vi "Start Sync.vi"(8 "error in (no error)":errorcluster, 11 "gRPC service in":refnum<class "OOBgRPCService.lvclass">) -> (0 "error out":errorcluster, 3 "gRPC service out":refnum<class "OOBgRPCService.lvclass">)   [LabVIEW 2025, in "OOB gRPC Server.lvlib" / "OOBgRPCService.lvclass"]
uses:
  OOBgRPCService.lvclass
  OOBgRPCService.lvclass/OOBgRPCService.ctl
  RPC Messages/hwval_GenericResponse.ctl
  RPC Messages/hwval_StatusResponse.ctl
  Dequeue Frame.vi
  OOB Data Transfer/OOB Data Transfer.lvlib
  OOB gRPC Server.lvlib
  CAN-LIN Raw Bus Capture.lvclass
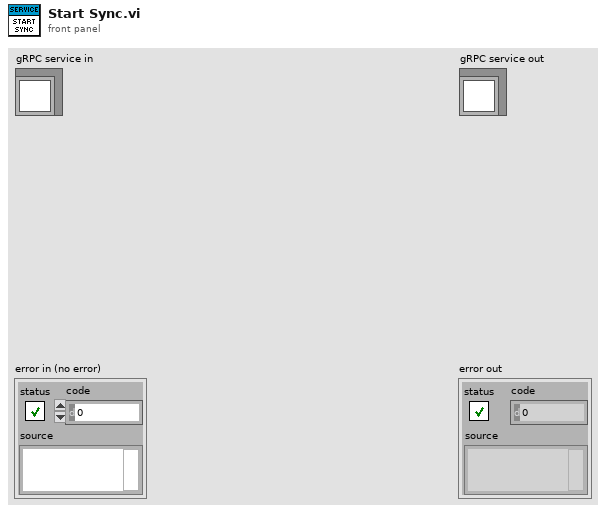
[diagram p1: front panel]
types:
  T1 = typedef "OOB gRPC Server.lvlib/hwval_GenericResponse.ctl" = cluster{"Payload":u8[]}
  T2 = typedef "OOB gRPC Server.lvlib/hwval_StatusResponse.ctl" = cluster{"Status":bool, "Code":i32, "Message":string}
  T3 = typedef "OOB gRPC Server.lvlib/OOBgRPCService.lvclass/Server Internal UEs.ctl" = cluster{"OOBgRPCService Generic Internal UE":refnum<user-event>, "OOBgRPCService PauseResume Internal UE":refnum<user-event>, "OOBgRPCService Export Internal UE":refnum<user-event>}
  T4 = typedef "OOB gRPC Server.lvlib/OOBgRPCService.lvclass/Server gRPC UEs.ctl" = cluster{"OOBgRPCService Generic gRPC UE":refnum<user-event>, "OOBgRPCService PauseResume gRPC UE":refnum<user-event>, "OOBgRPCService Export gRPC UE":refnum<user-event>}
  T5 = typedef "grpc-lvsupport-release.lvlib/grpcId.ctl" = u64
  T6 = typedef "OOB gRPC Server.lvlib/hwval_GenericRequest.ctl" = cluster{"Command":string, "Payload":u8[]}
  T7 = typedef "OOB Data Transfer.lvlib/OOB to Logic Data.ctl" = cluster{"PauseResume":bool, "Export":string}
  T8 = typedef "OOB gRPC Server.lvlib/hwval_BoolRequest.ctl" = cluster{"BooleanData":bool}
  T9 = typedef "OOB gRPC Server.lvlib/hwval_ExportRequest.ctl" = cluster{"FileType":string}
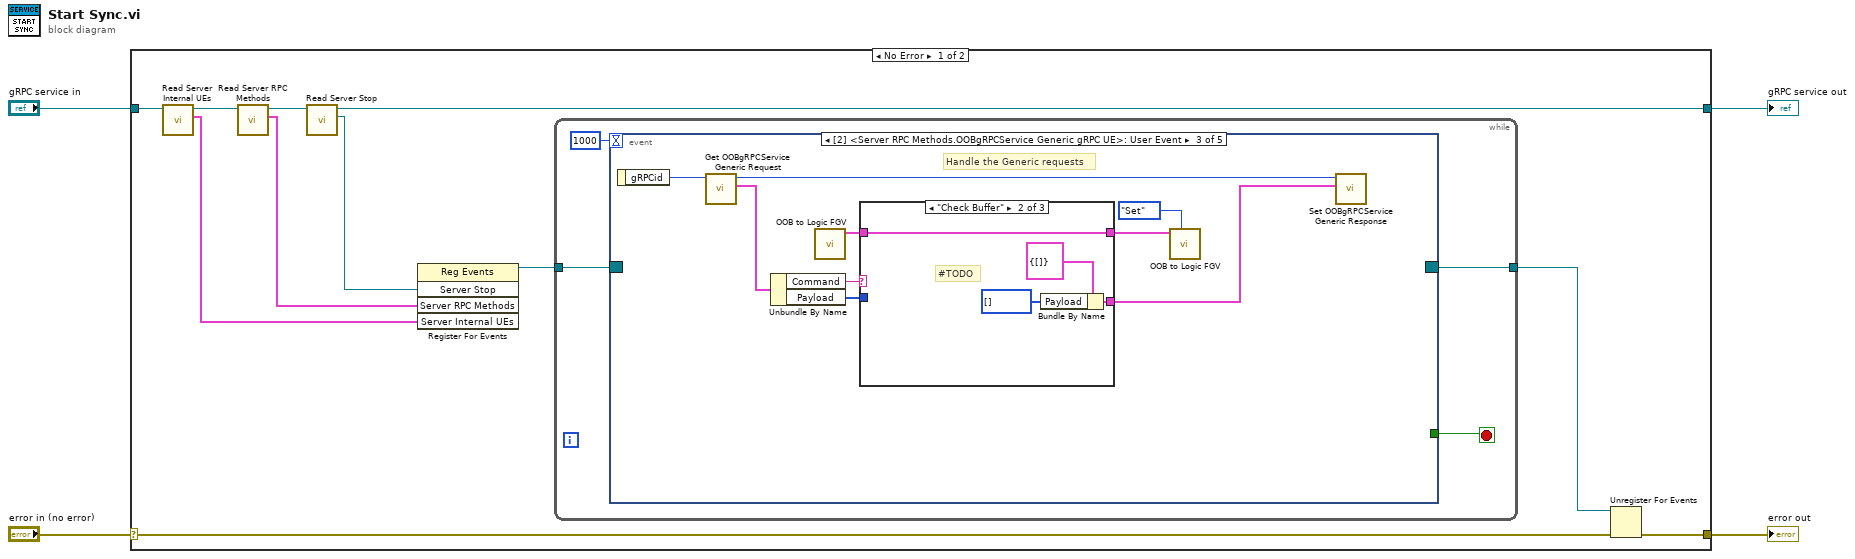
[diagram p0: block diagram]
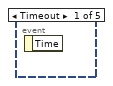
[diagram p2: hidden frame]
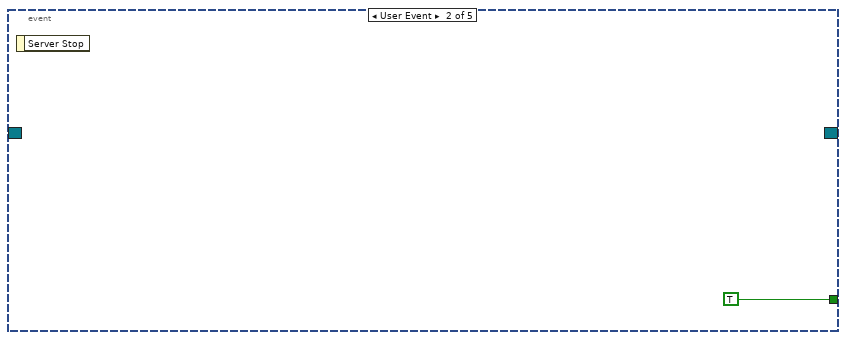
[diagram p3: hidden frame]
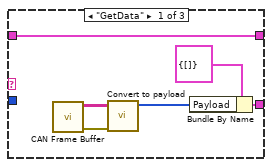
[diagram p4: hidden frame]
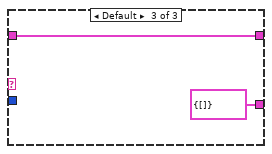
[diagram p5: hidden frame]
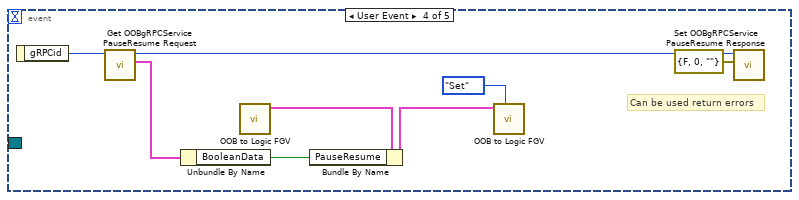
[diagram p6: hidden frame]
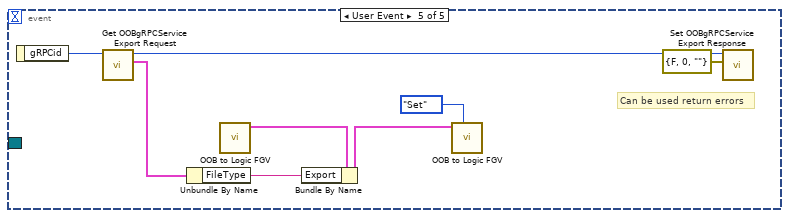
[diagram p7: hidden frame]
diagram:
  n1 = case shown="No Error" "error in (no error)" {
    selector: "error in (no error)" -> [w9 w59]
    tunnel: [w8 w59] -> w3
    tunnel: [w6 w58] -> w1
    tunnel: "gRPC service in" -> [w15 w58]
    frame No Error {
      n2 = call "Read Server Internal UEs.vi"("gRPC service in"=w15) -> ("Server Internal UEs"=w13:T3, "gRPC service out"=w14:refnum<class "OOBgRPCService.lvclass">)  [unwired: 8 in, 1 out]
      n3 = call "Read Server RPC Methods.vi"("gRPC service in"=w14) -> ("Server RPC Methods"=w7:T4, "gRPC service out"=w12:refnum<class "OOBgRPCService.lvclass">)  [unwired: 8 in, 1 out]
      n4 = call-dynamic "Read Server Stop.vi"("gRPC service in"=w12) -> ("Server Stop"=w5:refnum<user-event>, "gRPC service out"=w6:refnum<class "OOBgRPCService.lvclass">)  [unwired: 8 in, 1 out]
      n5 = register-events(w5, w7, w13) -> (reference out=w11:refnum<event-registration>)  [unwired: 2 in, 1 out]
      n6 = while {
        tunnel: w11 -> [w19]
        tunnel: [w17] -> w10
        stop <- w18 stop-if-true
        n7 = event "RPC Methods Event Structure" shown="[2] <Server RPC Methods.OOBgRPCService Generic gRPC UE>: User Event" {
          selector: w19 -> [_ _ _ _ _]
          dyn-events: [_ _ _ _ _] -> w17
          timeout: 1000 -> [_ _ _ _ _]
          tunnel: [_ TRUE _ _ _] -> w18
          event Timeout {
            n8 = event-data() -> ()  [unwired: 1 in, 1 out]
          }
          event User Event {
            n9 = event-data() -> ()  [unwired: 1 in, 1 out]
          }
          event User Event {
            # "Handle the Generic requests"
            n10 = event-data() -> ("gRPCid"=w29:T5)  [unwired: 1 in]
            n11 = call "Get OOBgRPCService Generic Request.vi"("gRPCid"=w29) -> ("Message Data"=w27:T6, "gRPCid out"=w28:T5)  [unwired: 8 in, 1 out]
            n12 = Unbundle By Name(w27) -> ("Command"=w23:string, "Payload"=w22:u8[])
            n13 = call "OOB to Logic FGV.vi"() -> ("OOB to Logic Data out"=w25:T7)  [unwired: 10 in, 1 out]
            n14 = case shown="\"Check Buffer\"" w23 {
              tunnel: w25 -> [w35 w39 w40]
              tunnel: [w35 w39 w40] -> w24
              tunnel: w22 -> [_ _ _]
              tunnel: [w31 w37 T1 {"Payload"=[]} ("Message Data")] -> w21
              frame "GetData" {
                n15 = call-poly "CAN Frame Buffer.vi"() -> ("error out"=w34:errorcluster, "Data"=w30:string[][])  [unwired: 10 in]
                n16 = call "Convert to payload.vi"("error in"=w34, "Data"=w30) -> ("U8 Array"=w32:u8[])  [unwired: 8 in, 1 out]
                n17 = Bundle By Name(cluster=T1 {"Payload"=[]} ("Message Data"), "Payload"=w32) -> (w31:T1)
              }
              frame "Check Buffer" {
                # "#TODO"
                n18 = Bundle By Name(cluster=T1 {"Payload"=[]} ("Message Data"), "Payload"=u8[] []) -> (w37:T1)
              }
              frame Default {
              }
            }
            n19 = call "OOB to Logic FGV.vi"("Op (Get)"=enum16{"Get", "Set"}."Set", "OOB to Logic Data in"=w24) -> ()  [unwired: 8 in, 2 out]
            n20 = call "Set OOBgRPCService Generic Response.vi"("Message Data"=w21, "gRPCid in"=w28) -> ()  [unwired: 9 in, 1 out]
          }
          event User Event {
            # "Can be used return errors"
            n21 = event-data() -> ("gRPCid"=w43:T5)  [unwired: 1 in]
            n22 = call "Get OOBgRPCService PauseResume Request.vi"("gRPCid"=w43) -> ("Message Data"=w45:T8, "gRPCid out"=w46:T5)  [unwired: 8 in, 1 out]
            n23 = Unbundle By Name(w45) -> ("BooleanData"=w44:bool)
            n24 = call "OOB to Logic FGV.vi"() -> ("OOB to Logic Data out"=w48:T7)  [unwired: 10 in, 1 out]
            n25 = Bundle By Name(cluster=w48, "PauseResume"=w44) -> (w47:T7)
            n26 = call "OOB to Logic FGV.vi"("Op (Get)"=enum16{"Get", "Set"}."Set", "OOB to Logic Data in"=w47) -> ()  [unwired: 8 in, 2 out]
            n27 = call "Set OOBgRPCService PauseResume Response.vi"("Message Data"=T2 {"Status"=FALSE, "Code"=0, "Message"=""}, "gRPCid in"=w46) -> ()  [unwired: 9 in, 1 out]
          }
          event User Event {
            # "Can be used return errors"
            n28 = event-data() -> ("gRPCid"=w51:T5)  [unwired: 1 in]
            n29 = call "Get OOBgRPCService Export Request.vi"("gRPCid"=w51) -> ("Message Data"=w53:T9, "gRPCid out"=w57:T5)  [unwired: 8 in, 1 out]
            n30 = Unbundle By Name(w53) -> ("FileType"=w52:string)
            n31 = call "OOB to Logic FGV.vi"() -> ("OOB to Logic Data out"=w55:T7)  [unwired: 10 in, 1 out]
            n32 = Bundle By Name(cluster=w55, "Export"=w52) -> (w54:T7)
            n33 = call "OOB to Logic FGV.vi"("Op (Get)"=enum16{"Get", "Set"}."Set", "OOB to Logic Data in"=w54) -> ()  [unwired: 8 in, 2 out]
            n34 = call "Set OOBgRPCService Export Response.vi"("Message Data"=T2 {"Status"=FALSE, "Code"=0, "Message"=""}, "gRPCid in"=w57) -> ()  [unwired: 9 in, 1 out]
          }
        }
      }
      n35 = Unregister For Events(event registration refnum=w10, error in=w9) -> (error out=w8:errorcluster)
    }
    frame Error {
    }
  }
  "error out" <- w3
  "gRPC service out" <- w1
